vi "ActivDesactivCtrlUSB.vi"(4 "error in (no error)":errorcluster, 6 "Disabled":T2(ring), 7 "ClusterRefCtrl_IN":T1) -> (0 "error out":errorcluster, 3 "ClusterRefCtrl_OUT":T1)   [LabVIEW 2017]
uses:
  DefDeType/ClusterRefCtrlUSBB.ctl
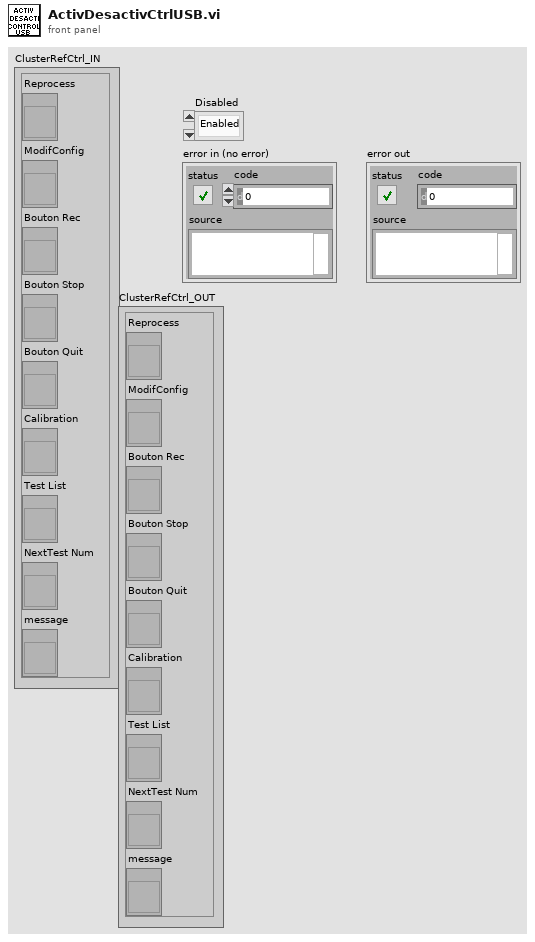
[diagram p1: front panel]
types:
  T1 = typedef "ClusterRefCtrlUSBB.ctl" = cluster{"Reprocess":refnum<vi>, "ModifConfig":refnum<vi>, "Bouton Rec":refnum<vi>, "Bouton Stop":refnum<vi>, "Bouton Quit":refnum<vi>, "Calibration":refnum<vi>, "Test List":refnum<vi>, "NextTest Num":refnum<vi>, "message":refnum<vi>}
  T2 = enum8{"Enabled", "Disabled", "Disabled and Grayed Out"}
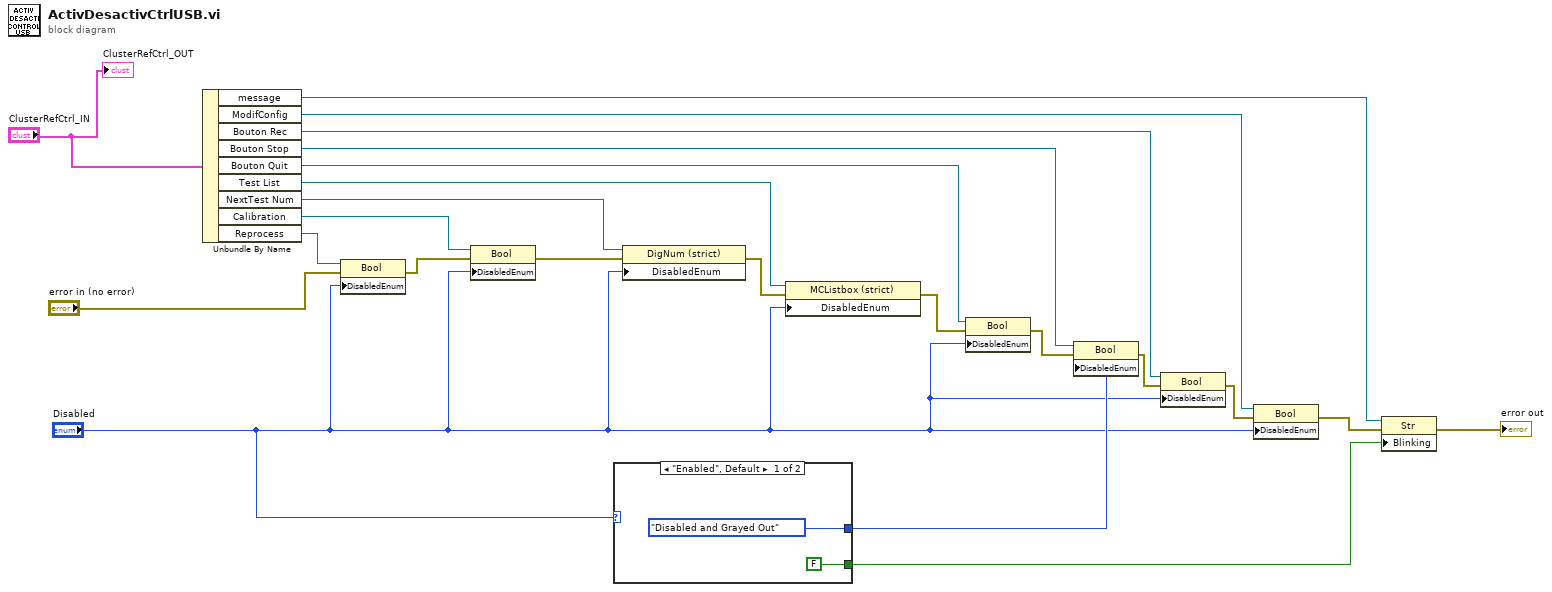
[diagram p0: block diagram]
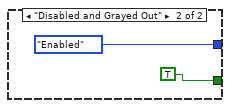
[diagram p2: hidden frame]
diagram:
  n1 = Unbundle By Name("ClusterRefCtrl_IN") -> ("message"=w11:refnum<vi>, "ModifConfig"=w16:refnum<vi>, "Bouton Rec"=w17:refnum<vi>, "Bouton Stop"=w18:refnum<vi>, "Bouton Quit"=w19:refnum<vi>, "Test List"=w20:refnum<vi>, "NextTest Num"=w21:refnum<vi>, "Calibration"=w7:refnum<vi>, "Reprocess"=w4:refnum<vi>)
  n2 = property class="Bool"(reference=w4, error in="error in (no error)", "DisabledEnum"="Disabled") -> (error out=w3:errorcluster)  [unwired: 1 out]
  n3 = property class="Bool"(reference=w7, error in=w3, "DisabledEnum"="Disabled") -> (error out=w6:errorcluster)  [unwired: 1 out]
  n4 = case shown="\"Enabled\", Default" "Disabled" {
    tunnel: [T2."Disabled and Grayed Out" ("Désactivé") T2."Enabled" ("Désactivé")] -> w12
    tunnel: [FALSE TRUE] -> w9
    frame "Enabled", Default {
    }
    frame "Disabled and Grayed Out" {
    }
  }
  n5 = property class="DigNum (strict)"(reference=w21, error in=w6, "DisabledEnum"="Disabled") -> (error out=w15:errorcluster)  [unwired: 1 out]
  n6 = property class="MCListbox (strict)"(reference=w20, error in=w15, "DisabledEnum"="Disabled") -> (error out=w14:errorcluster)  [unwired: 1 out]
  n7 = property class="Bool"(reference=w19, error in=w14, "DisabledEnum"="Disabled") -> (error out=w13:errorcluster)  [unwired: 1 out]
  n8 = property class="Bool"(reference=w18, error in=w13, "DisabledEnum"=w12) -> (error out=w22:errorcluster)  [unwired: 1 out]
  n9 = property class="Bool"(reference=w17, error in=w22, "DisabledEnum"="Disabled") -> (error out=w23:errorcluster)  [unwired: 1 out]
  n10 = property class="Bool"(reference=w16, error in=w23, "DisabledEnum"="Disabled") -> (error out=w10:errorcluster)  [unwired: 1 out]
  n11 = property class="Str"(reference=w11, error in=w10, "Blinking"=w9) -> (error out=→"error out":errorcluster)  [unwired: 1 out]
  "ClusterRefCtrl_OUT" <- "ClusterRefCtrl_IN"
